vi "Main.vi"() -> ()   [LabVIEW 2019]
uses:
  active object queue_class/active object queue.lvclass
  <vilib>/Platform/TimedLoop/XDataNode/timing_clust.ctl
  <vilib>/Platform/TimedLoop/XDataNode/nitl_modes.ctl
  <vilib>/Platform/TimedLoop/XDataNode/wakeup.ctl
  <vilib>/platform/TimedLoop/XDataNode/XDataNode.xnode
  <vilib>/Platform/TimedLoop/XDataNode/XDNodeRunTimeDep.lvlib
panel:
  out "Attribute":dbl
  out "Status":bool
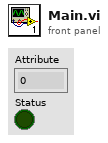
[diagram p1: front panel]
types:
  T1 = typedef "XDNodeRunTimeDep.lvlib/timing_clust.ctl" = cluster{"Expected End [f-1]":u64, "Actual End [f-1]":u64, "Finished Late? [f-1]":bool, "Expected End [i-1]":u64, "Actual End [i-1]":u64, "Finished Late? [i-1]":bool, "Expected Start [i]":u64, "Actual Start [i]":u64, "Expected Start [f]":u64, "Actual Start [f]":u64, "Source Name":string, "Structure Name":string, "Period":i64, "Deadline":i64, "Offset":i64, "Start":i64, "Priority":i32, "Timeout":i32, "Mode":T2, "Wakeup Reason":T3, "Error":errorcluster, "Source Type":string, "Secondary Source Type":string, "Global End Time":u64, "Global Start Time":u64, "Frame Duration":u64, "Iteration Duration":u64, "Assigned CPU":i32, "I/O Scan Engine Mode":u32}
  T2 = typedef "XDNodeRunTimeDep.lvlib/nitl_modes.ctl" = enum32{"No Change", "Process missed periods, maintain original phase", "Discard missed periods, maintain original phase", "Process missed periods, ignore original phase", "Discard missed periods, ignore original phase"}
  T3 = typedef "XDNodeRunTimeDep.lvlib/wakeup.ctl" = enum32{"Normal", "Aborted", "Asynchronous wakeup", "Timing source error", "Timed loop error", "Timeout"}
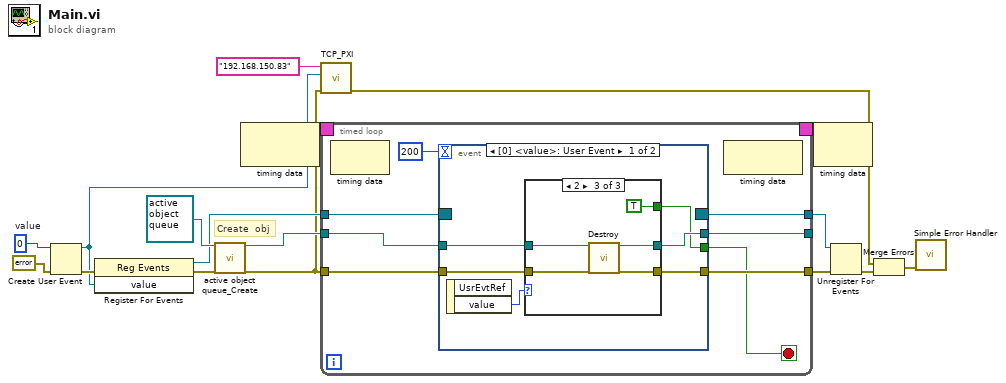
[diagram p0: block diagram]
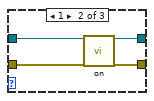
[diagram p3: hidden frame]
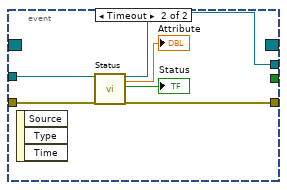
[diagram p4: hidden frame]
diagram:
  w16 = 0  # value
  # "Create  obj"
  n1 = Create User Event(user event datatype=w16, error in=errorcluster {"status"=FALSE, "code"=0, "source"=""} ("error out")) -> (user event=w9:refnum<user-event>, error out=w15:errorcluster)
  n2 = register-events(error in=w15, w9) -> (reference out=w14:refnum<event-registration>, error out=w3:errorcluster)  [unwired: 1 in]
  n3 = call "active object queue_Create.vi"("reference in"=refnum<class "active object queue.lvclass"> refnum ("active object queue"), "error in (no error)"=w3) -> ("reference out"=w13:refnum<class "active object queue.lvclass">, "error out"=w12:errorcluster)  [unwired: 16 in]
  n4 = node-c288() -> (w2:T1)  [unwired: 1 in]
  n5 = call "TCP_PXI.vi"("error in (no error) 2"=w12, "user event out"=w9, "Machine"="192.168.150.83") -> ("error out"=w8:errorcluster)  [unwired: 8 in]
  n6 = timed-loop {
    tunnel: w14 -> [w25]
    tunnel: w13 -> [w23]
    tunnel: w12 -> [w22]
    tunnel: [w21] -> _
    tunnel: [w20] -> w10
    tunnel: [w19] -> w11
    timing: w2 -> [_]
    timing-out: [_] -> w1
    stop <- w18 stop-if-true
    n7 = node-c288() -> ()  [unwired: 1 in, 1 out]
    n8 = event shown="[0] <value>: User Event" {
      selector: w25 -> [_ _]
      dyn-events: [_ _] -> w19
      timeout: 200 -> [_ _]
      tunnel: w23 -> [w32 w49]
      tunnel: w22 -> [w31 w48]
      tunnel: [w30 w47] -> w21
      tunnel: [w29 w46] -> w20
      tunnel: [w28 _] -> w18
      event User Event {
        n9 = event-data() -> ("value"=w33:i32)  [unwired: 1 in, 1 out]
        n10 = case shown="2" w33 {
          tunnel: [w35 w39 w43] -> w30
          tunnel: [w34 w38 w42] -> w29
          tunnel: w32 -> [w35 w37 w44]
          tunnel: w31 -> [w34 w36 w41]
          tunnel: [_ _ TRUE] -> w28
          frame 0, Default {
          }
          frame 1 {
            n11 = call "on.vi"("reference in"=w37, "error in (no error)"=w36) -> ("reference out"=w39:refnum<class "active object queue.lvclass">, "error out"=w38:errorcluster)  [unwired: 16 in]
          }
          frame 2 {
            n12 = call-dynamic "Destroy.vi"("reference in"=w44, "error in (no error)"=w41) -> ("reference out"=w43:refnum<class "active object queue.lvclass">, "error out"=w42:errorcluster)  [unwired: 16 in]
          }
        }
      }
      event Timeout {
        n13 = event-data() -> ()  [unwired: 1 in, 3 out]
        n14 = call-dynamic "Status.vi"("reference in"=w49, "error in (no error)"=w48) -> ("reference out"=w47:refnum<class "active object queue.lvclass">, "Attribute1"=→"Attribute":dbl, "Status"=→"Status":bool, "error out"=w46:errorcluster)  [unwired: 14 in]
      }
    }
    n15 = node-c288() -> ()  [unwired: 1 in, 1 out]
  }
  n16 = node-c288(w1) -> ()  [unwired: 1 out]
  n17 = Unregister For Events(event registration refnum=w11, error in=w10) -> (error out=w7:errorcluster)
  n18 = Merge Errors(w8, w7) -> (w6:errorcluster)
  n19 = call <vilib>:"Simple Error Handler.vi"("error in (no error)"=w6) -> ()  [unwired: 4 in, 5 out]
